vi "AudioTest.SoundCheck Data Log Graph Window - Composite.vi"() -> ()   [LabVIEW 2018]
uses:
  TypeDefs/AudioTest.Analysis Data Record.ctl
  <vilib>/KATE/Queues/Queue Utils.lvlib
panel:
  in  "Main Tab":enum32{"Data", "Setup"}(tab)
  in  "Snapshot":bool
  out "Name 1 1":string
  out "Graph1 1":cluster{"X":dbl[], "Y":dbl[]}[](graph)
  out "Graph1 2":cluster{"X":dbl[], "Y":dbl[]}[](graph)
  out "Name 1 2":string
  out "Name 3 3":string
  out "Graph3 3":cluster{"X":dbl[], "Y":dbl[]}[](graph)
  out "Name 3 2":string
  out "Graph3 2":cluster{"X":dbl[], "Y":dbl[]}[](graph)
  out "Name 3 1":string
  out "Graph3 1":cluster{"X":dbl[], "Y":dbl[]}[](graph)
  out "Name 2 4":string
  out "Graph2 4":cluster{"X":dbl[], "Y":dbl[]}[](graph)
  out "Graph2 3":cluster{"X":dbl[], "Y":dbl[]}[](graph)
  out "Name 2 3":string
  out "Graph2 2":cluster{"X":dbl[], "Y":dbl[]}[](graph)
  out "Name 2 2":string
  out "Graph2 1":cluster{"X":dbl[], "Y":dbl[]}[](graph)
  out "Name 2 1":string
  out "Graph1 4":cluster{"X":dbl[], "Y":dbl[]}[](graph)
  out "Name 1 4":string
  out "Graph1 3":cluster{"X":dbl[], "Y":dbl[]}[](graph)
  out "Name 1 3":string
  in  "Graphs":T1[](array[typedef])
  in  "QName":string="Plot_Composite"
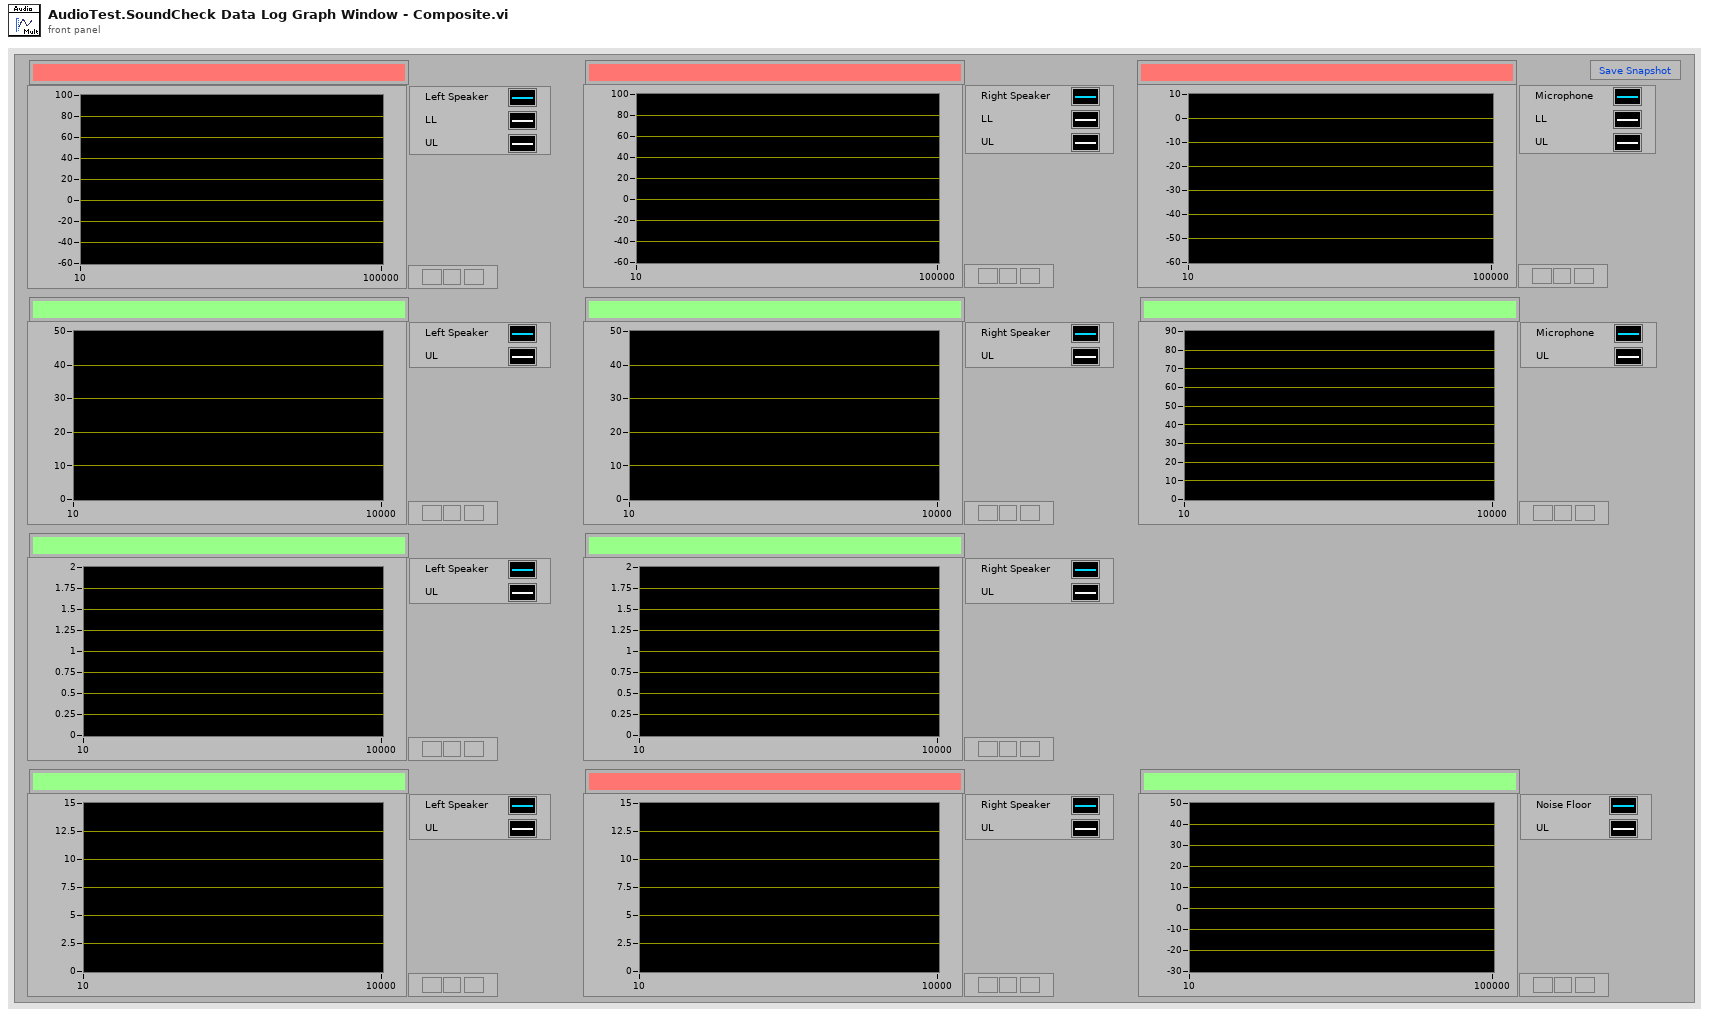
[diagram p1: front panel]
types:
  T1 = typedef "AudioTest.Analysis Data Record.ctl" = cluster{"Name":string, "X Units":string, "Y Units":string, "DataPlots":cluster{"X":dbl[], "Y":dbl[]}[], "LimitPlots":cluster{"X":dbl[], "Y":dbl[]}[], "DataPlotNames":string[], "LimitPlotNames":string[], "Fail":bool}
  T2 = typedef "imagedata.ctl" = cluster{"image type":i32, "image depth":i32, "image":u8[], "mask":u8[], "colors":u32[], "Rectangle":cluster{"left":i16, "top":i16, "right":i16, "bottom":i16}}
  T3 = enum32{"Invalid", "Standard", "Closed", "Hidden", "Minimized", "Maximized"}
  T4 = cluster{"Graphs":T1[], "PlotColors":u32[], "LimColors":u32[]}
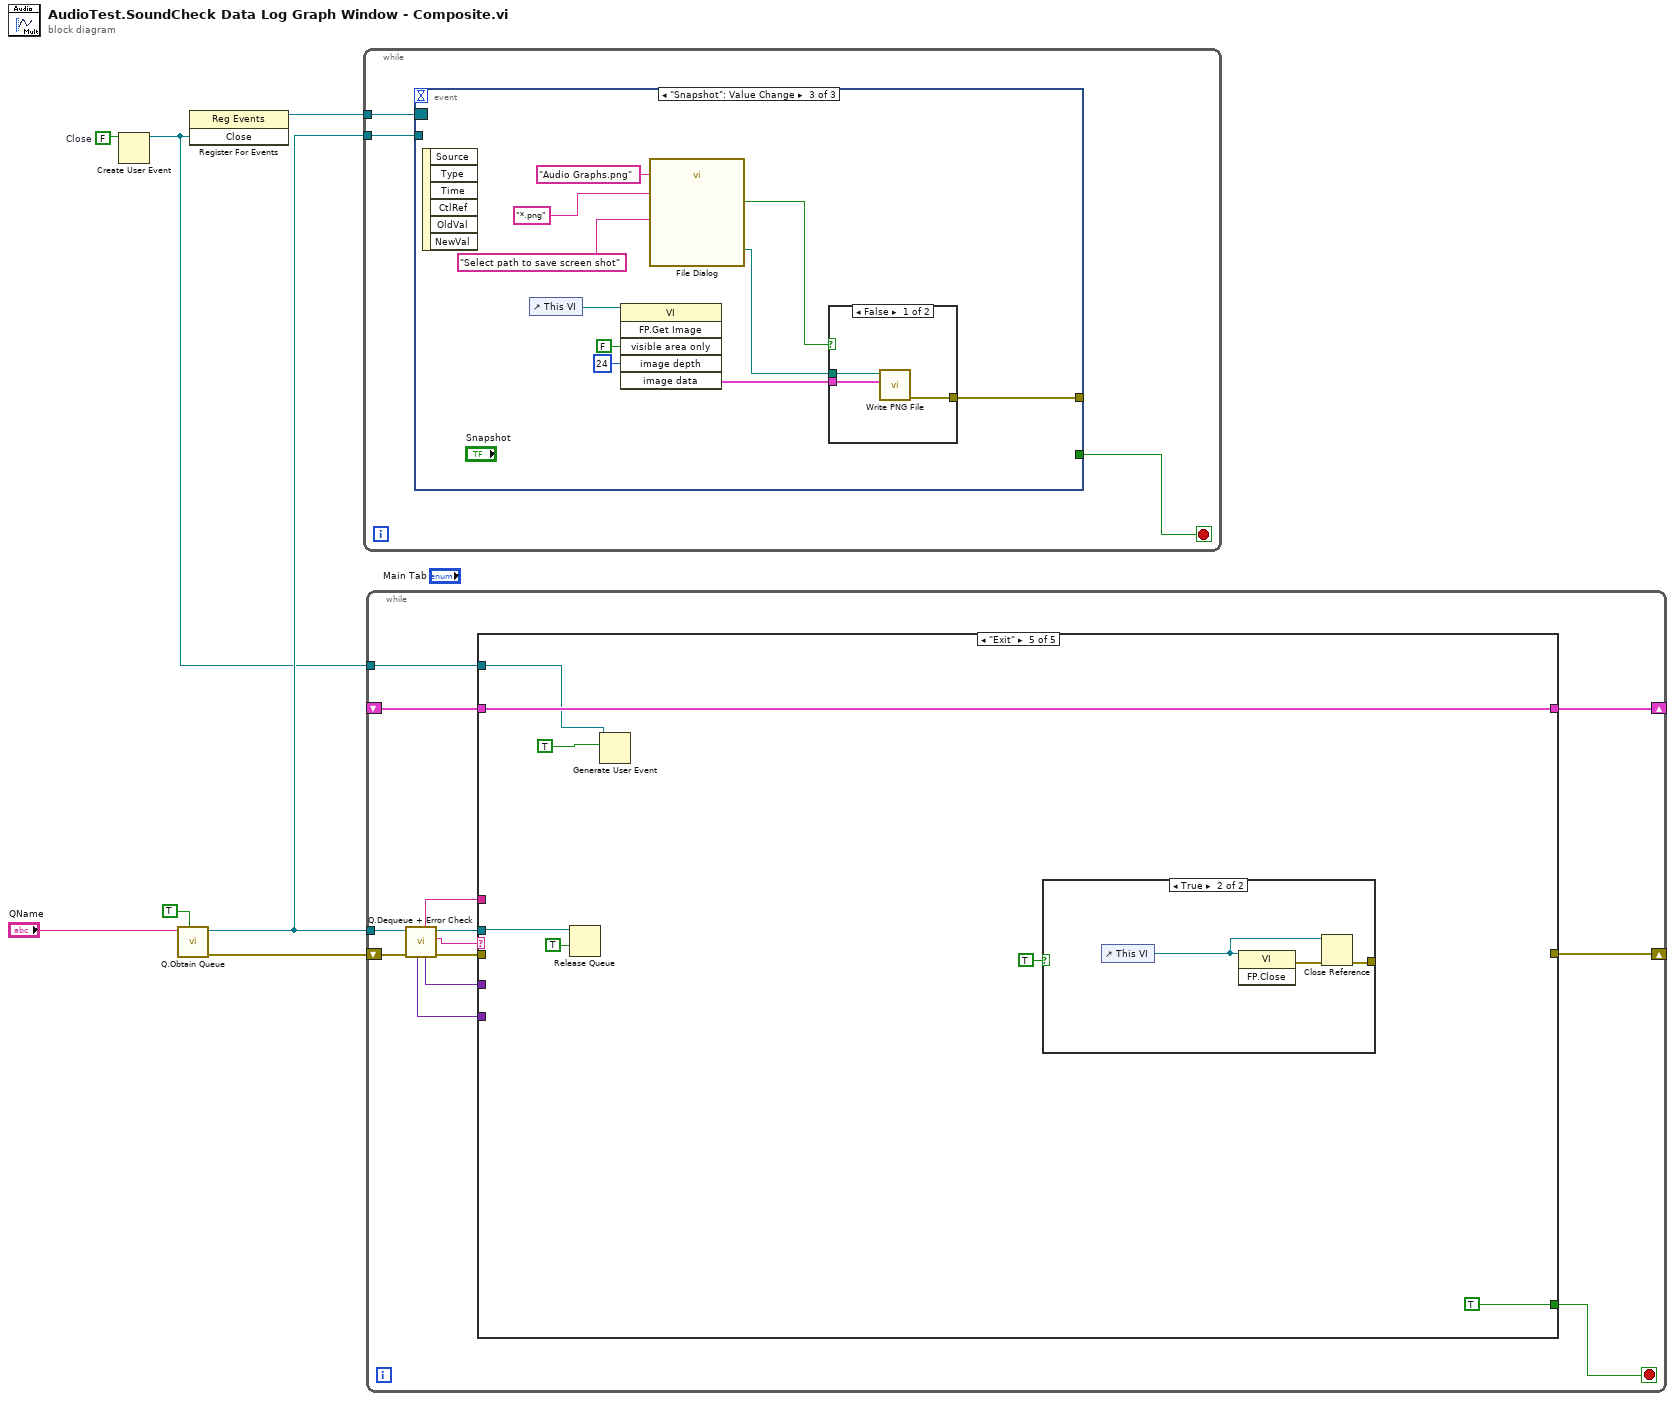
[diagram p0: block diagram]
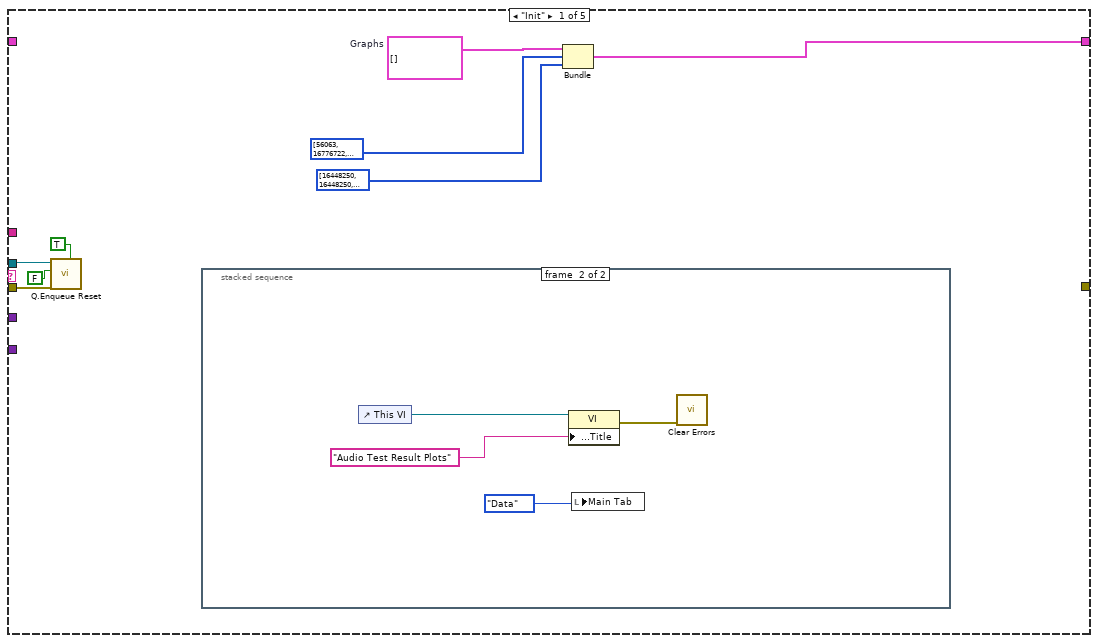
[diagram p2: hidden frame]
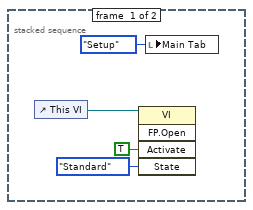
[diagram p3: hidden frame]
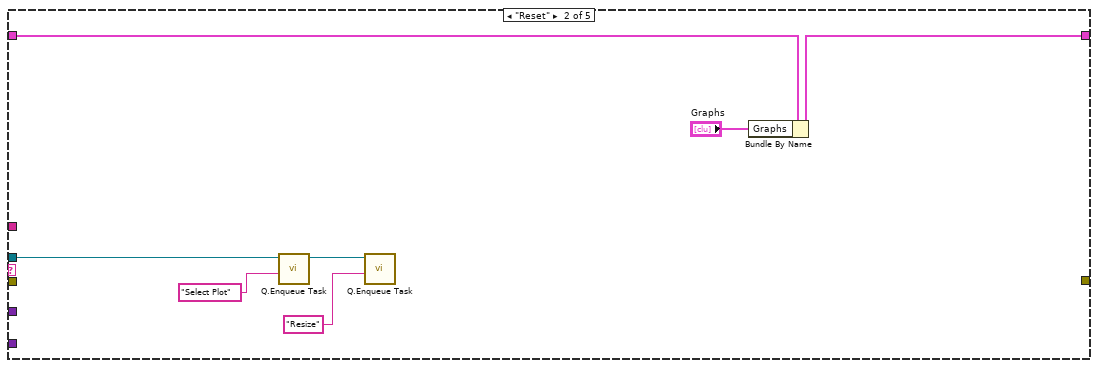
[diagram p4: hidden frame]
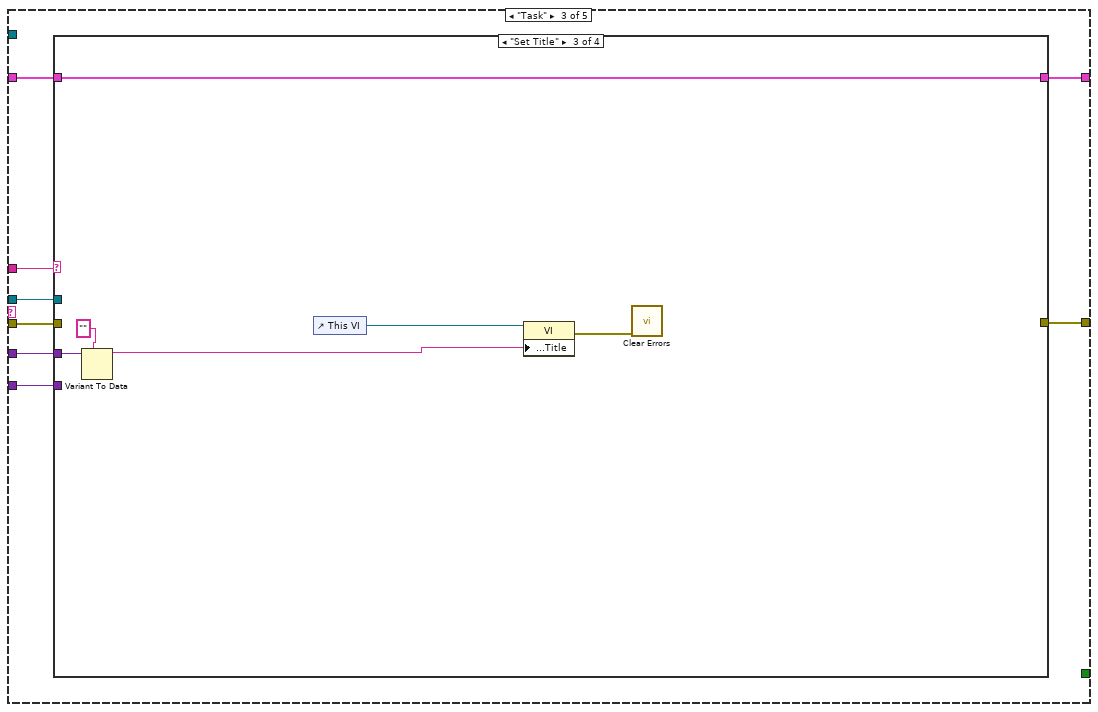
[diagram p5: hidden frame]
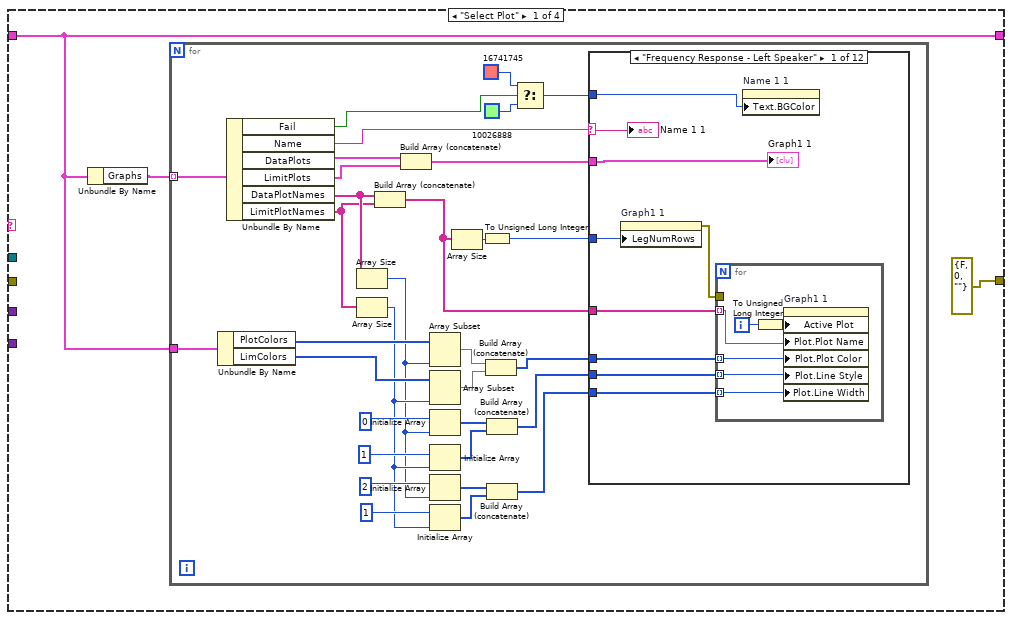
[diagram p6: hidden frame]
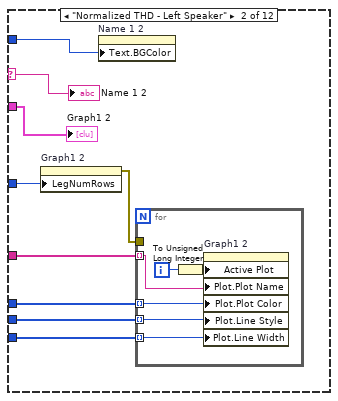
[diagram p7: hidden frame]
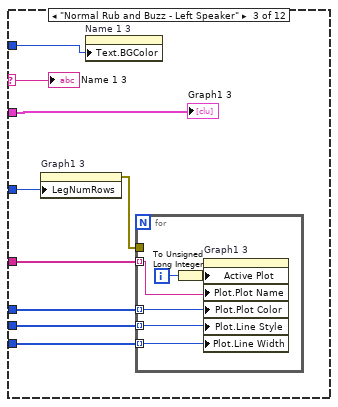
[diagram p8: hidden frame]
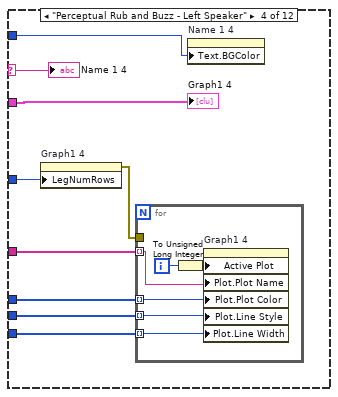
[diagram p9: hidden frame]
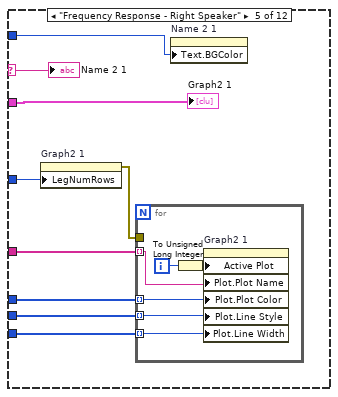
[diagram p10: hidden frame]
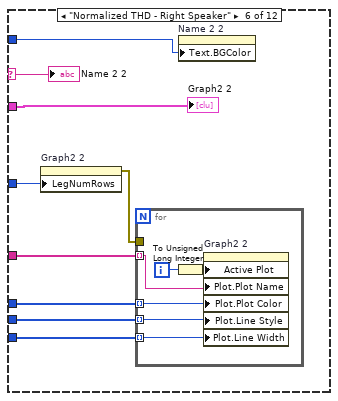
[diagram p11: hidden frame]
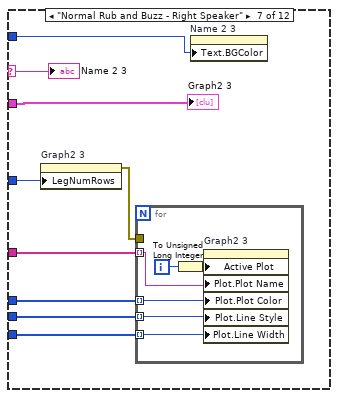
[diagram p12: hidden frame]
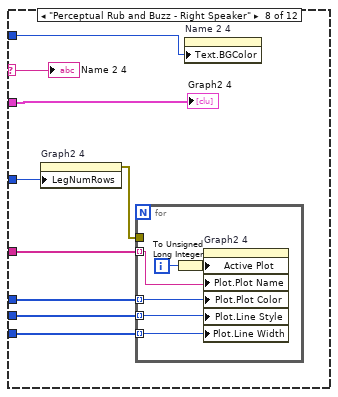
[diagram p13: hidden frame]
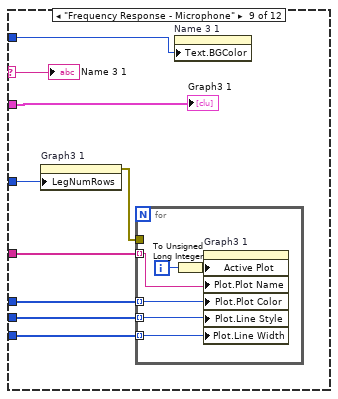
[diagram p14: hidden frame]
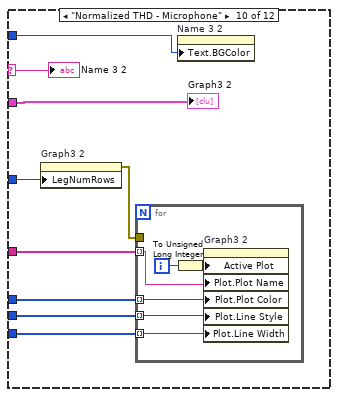
[diagram p15: hidden frame]
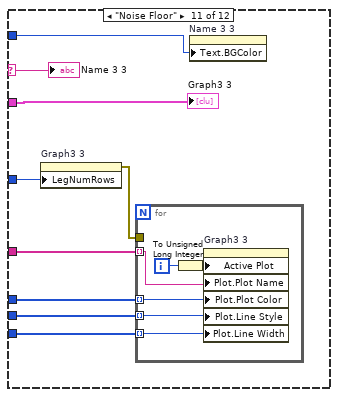
[diagram p16: hidden frame]
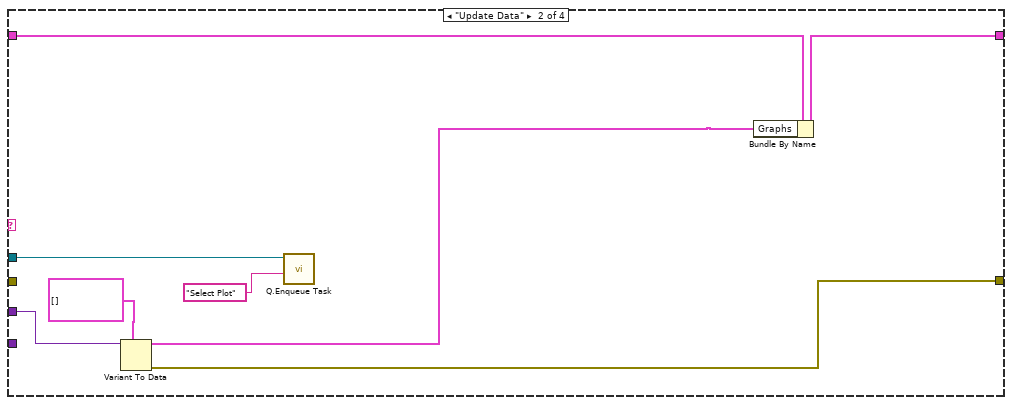
[diagram p18: hidden frame]
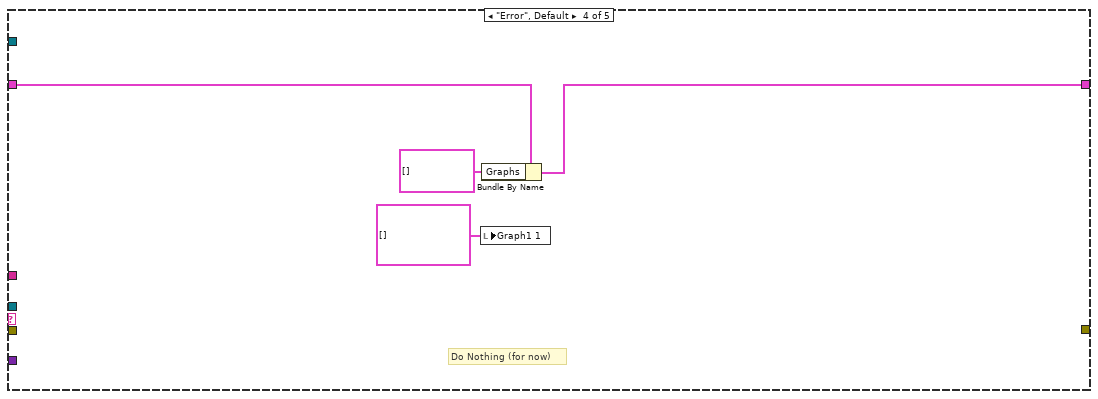
[diagram p20: hidden frame]
diagram:
  w7 = FALSE  # Close
  n1 = Create User Event(user event datatype=w7) -> (user event=w2:refnum<user-event>)  [unwired: 1 in, 1 out]
  n2 = call <vilib>:"Q.Obtain Queue.vi"("Enqueue Init"=TRUE, "Q Name"="QName") -> ("error out"=w4:errorcluster, "Q Out"=w3:refnum<queue>)  [unwired: 7 in, 1 out]
  n3 = register-events(w2) -> (reference out=w6:refnum<event-registration>)  [unwired: 2 in, 1 out]
  n4 = while {
    tunnel: w6 -> [w10]
    tunnel: w3 -> [w9]
    stop <- w8 stop-if-true
    n5 = event shown="[2] \"Snapshot\": Value Change" {
      selector: w10 -> [_ _ _]
      dyn-events: _ -> [_ _ _]
      timeout: _ -> [_ _ _]
      tunnel: w9 -> [w13 w16 _]
      tunnel: [TRUE TRUE _] -> w8
      tunnel: [_ _ w23] -> _
      event Panel Close? {
        n6 = event-data() -> ()  [unwired: 1 in, 4 out]
        n7 = call <vilib>:"Q.Enqueue Exit.vi"("Q In"=w13) -> ("error out"=w12:errorcluster)  [unwired: 9 in, 1 out]
        n8 = call <vilib>:"Clear Errors.vi"("error in (no error)"=w12) -> ()  [unwired: 5 in, 2 out]
        n9 = event-data("Discard?"=TRUE) -> ()  [unwired: 1 in, 1 out]
      }
      event User Event {
        n10 = event-data() -> ()  [unwired: 1 in, 4 out]
        n11 = call <vilib>:"Q.Enqueue Exit.vi"("Q In"=w16) -> ("error out"=w15:errorcluster)  [unwired: 9 in, 1 out]
        n12 = call <vilib>:"Clear Errors.vi"("error in (no error)"=w15) -> ()  [unwired: 5 in, 2 out]
      }
      event "Snapshot": Value Change {
        n13 = event-data() -> ()  [unwired: 1 in, 6 out]
        n14 = control-ref of="This VI"() -> (w27:refnum<vi>)
        n15 = invoke class="VI" method="FP.Get Image"(reference=w27, "visible area only"=FALSE ("Visible Area Only"), "image depth"=24 ("Image Depth")) -> ("image data"=w24:T2)  [unwired: 3 in, 5 out]
        n16 = call "File Dialog"("prompt"="Select path to save screen shot", "default name"="Audio Graphs.png", "pattern (all files)"="*.png") -> ("selected path"=w22:path, "cancelled"=w18:bool)  [unwired: 9 in, 2 out]
        n17 = case shown="False" w18 {
          tunnel: w24 -> [w30 _]
          tunnel: [w29 _] -> w23
          tunnel: w22 -> [w28 _]
          frame False {
            n18 = call <vilib>:"Write PNG File.vi"("image data"=w30, "path to PNG file"=w28) -> ("error out"=w29:errorcluster)  [unwired: 8 in, 1 out]
          }
          frame True {
          }
        }
      }
    }
  }
  n19 = while {
    shift-right: [w35] -> _
    shift-left: w4 -> [w40]
    tunnel: w3 -> [w38]
    shift-right: [w33] -> _
    shift-left: _ -> [w32]
    tunnel: w2 -> [w31]
    stop <- w34 stop-if-true
    n20 = call <vilib>:"Q.Dequeue + Error Check.vi"("Error In"=w40, "Q In"=w38) -> ("error out"=w41:errorcluster, "Cmd"=w43:string, "Q Out"=w42:refnum<queue>, "Data1"=w37:variant, "Sub"=w39:string, "Data2"=w36:variant)  [unwired: 4 in]
    n21 = case shown="\"Exit\"" w43 {
      tunnel: w42 -> [w51 w64 w73 _ w295]
      tunnel: w41 -> [w50 _ w72 _ _]
      tunnel: w39 -> [_ _ w74 _ _]
      tunnel: w37 -> [_ _ w71 _ _]
      tunnel: w36 -> [_ _ w70 _ _]
      tunnel: [_ _ w67 _ _] -> w35
      tunnel: [_ _ _ _ TRUE] -> w34
      tunnel: [w45 w66 w68 w292 w299] -> w33
      tunnel: w32 -> [_ w65 w69 w293 w299]
      tunnel: w31 -> [_ _ _ _ w298]
      frame "Init" {
        w48 = T1[] []  # Graphs
        n22 = call <vilib>:"Q.Enqueue Reset.vi"("Top of Q(T)"=TRUE, "Error In"=w50, "Flush Queue(T)"=FALSE, "Q In"=w51) -> ()  [unwired: 6 in, 2 out]
        n23 = stacked-sequence {
          frame #0 {
            n24 = control-ref of="This VI"() -> (w55:refnum<vi>)
            n25 = invoke class="VI" method="FP.Open"(reference=w55, "Activate"=TRUE ("Activate?"), "State"=T3."Standard") -> ()  [unwired: 2 in, 5 out]
            n26 = local write "Main Tab"(enum32{"Data", "Setup"}."Setup" ("Main Tab")) -> ()
          }
          frame #1 {
            n27 = control-ref of="This VI"() -> (w59:refnum<vi>)
            n28 = property class="VI"(reference=w59, "Front Panel.Title"="Audio Test Result Plots") -> (error out=w58:errorcluster)  [unwired: 1 in, 1 out]
            n29 = local write "Main Tab"(enum32{"Data", "Setup"}."Data" ("Main Tab")) -> ()
            n30 = call <vilib>:"Clear Errors.vi"("error in (no error)"=w58) -> ()  [unwired: 5 in, 2 out]
          }
        }
        n31 = Bundle("Graphs"=w48, "PlotColors"=u32[] [56063, 16776722, 16730898, 16711925, 6618880], "LimColors"=u32[] [16448250, 16448250, 16448250, 16448250, 16448250, 16448250]) -> (w45:T4)  [unwired: 1 in]
      }
      frame "Reset" {
        n32 = call <vilib>:"Q.Enqueue Task.vi"("Task Name"="Select Plot", "Q In"=w64) -> ("Q Out"=w61:refnum<queue>)  [unwired: 8 in, 1 out]
        n33 = call <vilib>:"Q.Enqueue Task.vi"("Task Name"="Resize", "Q In"=w61) -> ()  [unwired: 8 in, 2 out]
        n34 = Bundle By Name(cluster=w65, "Graphs"="Graphs") -> (w66:T4)
      }
      frame "Task" {
        n35 = case shown="\"Set Title\"" w74 {
          tunnel: w73 -> [_ w281 _ _]
          tunnel: w72 -> [_ _ _ _]
          tunnel: w71 -> [_ w278 w285 _]
          tunnel: w70 -> [_ _ _ _]
          tunnel: w69 -> [w77 w280 w288 w289]
          tunnel: [w77 w279 w288 w289] -> w68
          tunnel: [errorcluster {"status"=FALSE, "code"=0, "source"=""} ("error constant") w277 _ _] -> w67
          frame "Select Plot" {
            n36 = Unbundle By Name(w77) -> ("Graphs"=w75:T1[])
            n37 = for {
              tunnel: w77 -> [w104]
              tunnel: w75 -> [w83] mode=indexing
              n38 = Unbundle By Name(w104) -> ("PlotColors"=w101:u32[], "LimColors"=w100:u32[])
              n39 = Unbundle By Name(w83) -> ("Fail"=w79:bool, "Name"=w82:string, "DataPlots"=w109:cluster{"X":dbl[], "Y":dbl[]}[], "LimitPlots"=w108:cluster{"X":dbl[], "Y":dbl[]}[], "DataPlotNames"=w103:string[], "LimitPlotNames"=w102:string[])
              n40 = Array Size(array=w103) -> (size(s)=w86:i32)
              n41 = Array Size(array=w102) -> (size(s)=w87:i32)
              n42 = Build Array (concatenate)(w103, w102) -> (w105:string[])
              n43 = Build Array (concatenate)(w109, w108) -> (w84:cluster{"X":dbl[], "Y":dbl[]}[])
              n44 = Array Subset(array=w101, length=w86) -> (w99:u32[])  [unwired: 1 in]
              n45 = Array Subset(array=w100, length=w87) -> (w98:u32[])  [unwired: 1 in]
              n46 = Initialize Array(u8 0 ("Plot.Line Style"), w86) -> (w94:u8[])
              n47 = Initialize Array(u8 1 ("Plot.Line Style"), w87) -> (w93:u8[])
              n48 = Initialize Array(u8 2 ("Plot.Line Style"), w86) -> (w90:u8[])
              n49 = Initialize Array(u8 1 ("Plot.Line Style"), w87) -> (w91:u8[])
              n50 = Array Size(array=w105) -> (size(s)=w107:i32)
              n51 = To Unsigned Long Integer(number=w107) -> (unsigned 32bit integer=w106:u32)
              n52 = Build Array (concatenate)(w99, w98) -> (w97:u32[])
              n53 = Build Array (concatenate)(w94, w93) -> (w92:u8[])
              n54 = Build Array (concatenate)(w90, w91) -> (w85:u8[])
              n55 = Select(t=u32 16741745, s=w79, f=u32 10026888) -> (s? t:f=w78:u32)
              n56 = case shown="\"Frequency Response - Left Speaker\"" w82 {
                selector: w82 -> [w111 w126 w141 w156 w171 w186 w201 w216 w231 w246 w261 _]
                tunnel: w106 -> [w118 w133 w148 w163 w178 w193 w208 w223 w238 w253 w268 _]
                tunnel: w105 -> [w116 w131 w146 w161 w176 w191 w206 w221 w236 w251 w266 _]
                tunnel: w97 -> [w115 w130 w145 w160 w175 w190 w205 w220 w235 w250 w265 _]
                tunnel: w92 -> [w114 w129 w144 w159 w174 w189 w204 w219 w234 w249 w264 _]
                tunnel: w85 -> [w113 w128 w143 w158 w173 w188 w203 w218 w233 w248 w263 _]
                tunnel: w84 -> [w112 w127 w142 w157 w172 w187 w202 w217 w232 w247 w262 _]
                tunnel: w78 -> [w110 w125 w140 w155 w170 w185 w200 w215 w230 w245 w260 _]
                frame "Frequency Response - Left Speaker" {
                  n57 = property on="Graph1 1" class="XYGraph (strict)"("LegNumRows"=w118) -> (error out=w117:errorcluster)  [unwired: 2 in, 1 out]
                  n58 = for {
                    tunnel: w116 -> [w122] mode=indexing
                    tunnel: w117 -> [_]
                    tunnel: w115 -> [w121] mode=indexing
                    tunnel: w114 -> [w120] mode=indexing
                    tunnel: w113 -> [w119] mode=indexing
                    i -> [w123]
                    n59 = To Unsigned Long Integer(number=w123) -> (unsigned 32bit integer=w124:u32)
                    n60 = property on="Graph1 1" class="XYGraph (strict)"("Active Plot"=w124, "Plot.Plot Name"=w122, "Plot.Plot Color"=w121, "Plot.Line Style"=w120, "Plot.Line Width"=w119) -> ()  [unwired: 2 in, 2 out]
                  }
                  n61 = property on="Name 1 1" class="Str"("Text.BGColor"=w110) -> ()  [unwired: 2 in, 2 out]
                  "Graph1 1" <- w112
                  "Name 1 1" <- w111
                }
                frame "Normalized THD - Left Speaker" {
                  n62 = property on="Graph1 2" class="XYGraph (strict)"("LegNumRows"=w133) -> (error out=w132:errorcluster)  [unwired: 2 in, 1 out]
                  n63 = property on="Name 1 2" class="Str"("Text.BGColor"=w125) -> ()  [unwired: 2 in, 2 out]
                  n64 = for {
                    tunnel: w131 -> [w137] mode=indexing
                    tunnel: w132 -> [_]
                    tunnel: w130 -> [w136] mode=indexing
                    tunnel: w129 -> [w135] mode=indexing
                    tunnel: w128 -> [w134] mode=indexing
                    i -> [w138]
                    n65 = To Unsigned Long Integer(number=w138) -> (unsigned 32bit integer=w139:u32)
                    n66 = property on="Graph1 2" class="XYGraph (strict)"("Active Plot"=w139, "Plot.Plot Name"=w137, "Plot.Plot Color"=w136, "Plot.Line Style"=w135, "Plot.Line Width"=w134) -> ()  [unwired: 2 in, 2 out]
                  }
                  "Graph1 2" <- w127
                  "Name 1 2" <- w126
                }
                frame "Normal Rub and Buzz - Left Speaker" {
                  n67 = property on="Graph1 3" class="XYGraph (strict)"("LegNumRows"=w148) -> (error out=w147:errorcluster)  [unwired: 2 in, 1 out]
                  n68 = property on="Name 1 3" class="Str"("Text.BGColor"=w140) -> ()  [unwired: 2 in, 2 out]
                  n69 = for {
                    tunnel: w146 -> [w152] mode=indexing
                    tunnel: w147 -> [_]
                    tunnel: w145 -> [w151] mode=indexing
                    tunnel: w144 -> [w150] mode=indexing
                    tunnel: w143 -> [w149] mode=indexing
                    i -> [w153]
                    n70 = To Unsigned Long Integer(number=w153) -> (unsigned 32bit integer=w154:u32)
                    n71 = property on="Graph1 3" class="XYGraph (strict)"("Active Plot"=w154, "Plot.Plot Name"=w152, "Plot.Plot Color"=w151, "Plot.Line Style"=w150, "Plot.Line Width"=w149) -> ()  [unwired: 2 in, 2 out]
                  }
                  "Graph1 3" <- w142
                  "Name 1 3" <- w141
                }
                frame "Perceptual Rub and Buzz - Left Speaker" {
                  n72 = property on="Graph1 4" class="XYGraph (strict)"("LegNumRows"=w163) -> (error out=w162:errorcluster)  [unwired: 2 in, 1 out]
                  n73 = for {
                    tunnel: w161 -> [w167] mode=indexing
                    tunnel: w162 -> [_]
                    tunnel: w160 -> [w166] mode=indexing
                    tunnel: w159 -> [w165] mode=indexing
                    tunnel: w158 -> [w164] mode=indexing
                    i -> [w168]
                    n74 = To Unsigned Long Integer(number=w168) -> (unsigned 32bit integer=w169:u32)
                    n75 = property on="Graph1 4" class="XYGraph (strict)"("Active Plot"=w169, "Plot.Plot Name"=w167, "Plot.Plot Color"=w166, "Plot.Line Style"=w165, "Plot.Line Width"=w164) -> ()  [unwired: 2 in, 2 out]
                  }
                  n76 = property on="Name 1 4" class="Str"("Text.BGColor"=w155) -> ()  [unwired: 2 in, 2 out]
                  "Graph1 4" <- w157
                  "Name 1 4" <- w156
                }
                frame "Frequency Response - Right Speaker" {
                  n77 = property on="Graph2 1" class="XYGraph (strict)"("LegNumRows"=w178) -> (error out=w177:errorcluster)  [unwired: 2 in, 1 out]
                  n78 = for {
                    tunnel: w176 -> [w182] mode=indexing
                    tunnel: w177 -> [_]
                    tunnel: w175 -> [w181] mode=indexing
                    tunnel: w174 -> [w180] mode=indexing
                    tunnel: w173 -> [w179] mode=indexing
                    i -> [w183]
                    n79 = To Unsigned Long Integer(number=w183) -> (unsigned 32bit integer=w184:u32)
                    n80 = property on="Graph2 1" class="XYGraph (strict)"("Active Plot"=w184, "Plot.Plot Name"=w182, "Plot.Plot Color"=w181, "Plot.Line Style"=w180, "Plot.Line Width"=w179) -> ()  [unwired: 2 in, 2 out]
                  }
                  n81 = property on="Name 2 1" class="Str"("Text.BGColor"=w170) -> ()  [unwired: 2 in, 2 out]
                  "Graph2 1" <- w172
                  "Name 2 1" <- w171
                }
                frame "Normalized THD - Right Speaker" {
                  n82 = property on="Graph2 2" class="XYGraph (strict)"("LegNumRows"=w193) -> (error out=w192:errorcluster)  [unwired: 2 in, 1 out]
                  n83 = for {
                    tunnel: w191 -> [w197] mode=indexing
                    tunnel: w192 -> [_]
                    tunnel: w190 -> [w196] mode=indexing
                    tunnel: w189 -> [w195] mode=indexing
                    tunnel: w188 -> [w194] mode=indexing
                    i -> [w198]
                    n84 = To Unsigned Long Integer(number=w198) -> (unsigned 32bit integer=w199:u32)
                    n85 = property on="Graph2 2" class="XYGraph (strict)"("Active Plot"=w199, "Plot.Plot Name"=w197, "Plot.Plot Color"=w196, "Plot.Line Style"=w195, "Plot.Line Width"=w194) -> ()  [unwired: 2 in, 2 out]
                  }
                  n86 = property on="Name 2 2" class="Str"("Text.BGColor"=w185) -> ()  [unwired: 2 in, 2 out]
                  "Graph2 2" <- w187
                  "Name 2 2" <- w186
                }
                frame "Normal Rub and Buzz - Right Speaker" {
                  n87 = property on="Graph2 3" class="XYGraph (strict)"("LegNumRows"=w208) -> (error out=w207:errorcluster)  [unwired: 2 in, 1 out]
                  n88 = for {
                    tunnel: w206 -> [w212] mode=indexing
                    tunnel: w207 -> [_]
                    tunnel: w205 -> [w211] mode=indexing
                    tunnel: w204 -> [w210] mode=indexing
                    tunnel: w203 -> [w209] mode=indexing
                    i -> [w213]
                    n89 = To Unsigned Long Integer(number=w213) -> (unsigned 32bit integer=w214:u32)
                    n90 = property on="Graph2 3" class="XYGraph (strict)"("Active Plot"=w214, "Plot.Plot Name"=w212, "Plot.Plot Color"=w211, "Plot.Line Style"=w210, "Plot.Line Width"=w209) -> ()  [unwired: 2 in, 2 out]
                  }
                  n91 = property on="Name 2 3" class="Str"("Text.BGColor"=w200) -> ()  [unwired: 2 in, 2 out]
                  "Graph2 3" <- w202
                  "Name 2 3" <- w201
                }
                frame "Perceptual Rub and Buzz - Right Speaker" {
                  n92 = property on="Graph2 4" class="XYGraph (strict)"("LegNumRows"=w223) -> (error out=w222:errorcluster)  [unwired: 2 in, 1 out]
                  n93 = for {
                    tunnel: w221 -> [w227] mode=indexing
                    tunnel: w222 -> [_]
                    tunnel: w220 -> [w226] mode=indexing
                    tunnel: w219 -> [w225] mode=indexing
                    tunnel: w218 -> [w224] mode=indexing
                    i -> [w228]
                    n94 = To Unsigned Long Integer(number=w228) -> (unsigned 32bit integer=w229:u32)
                    n95 = property on="Graph2 4" class="XYGraph (strict)"("Active Plot"=w229, "Plot.Plot Name"=w227, "Plot.Plot Color"=w226, "Plot.Line Style"=w225, "Plot.Line Width"=w224) -> ()  [unwired: 2 in, 2 out]
                  }
                  n96 = property on="Name 2 4" class="Str"("Text.BGColor"=w215) -> ()  [unwired: 2 in, 2 out]
                  "Graph2 4" <- w217
                  "Name 2 4" <- w216
                }
                frame "Frequency Response - Microphone" {
                  n97 = property on="Graph3 1" class="XYGraph (strict)"("LegNumRows"=w238) -> (error out=w237:errorcluster)  [unwired: 2 in, 1 out]
                  n98 = for {
                    tunnel: w236 -> [w242] mode=indexing
                    tunnel: w237 -> [_]
                    tunnel: w235 -> [w241] mode=indexing
                    tunnel: w234 -> [w240] mode=indexing
                    tunnel: w233 -> [w239] mode=indexing
                    i -> [w243]
                    n99 = To Unsigned Long Integer(number=w243) -> (unsigned 32bit integer=w244:u32)
                    n100 = property on="Graph3 1" class="XYGraph (strict)"("Active Plot"=w244, "Plot.Plot Name"=w242, "Plot.Plot Color"=w241, "Plot.Line Style"=w240, "Plot.Line Width"=w239) -> ()  [unwired: 2 in, 2 out]
                  }
                  n101 = property on="Name 3 1" class="Str"("Text.BGColor"=w230) -> ()  [unwired: 2 in, 2 out]
                  "Graph3 1" <- w232
                  "Name 3 1" <- w231
                }
                frame "Normalized THD - Microphone" {
                  n102 = property on="Graph3 2" class="XYGraph (strict)"("LegNumRows"=w253) -> (error out=w252:errorcluster)  [unwired: 2 in, 1 out]
                  n103 = for {
                    tunnel: w251 -> [w257] mode=indexing
                    tunnel: w252 -> [_]
                    tunnel: w250 -> [w256] mode=indexing
                    tunnel: w249 -> [w255] mode=indexing
                    tunnel: w248 -> [w254] mode=indexing
                    i -> [w258]
                    n104 = To Unsigned Long Integer(number=w258) -> (unsigned 32bit integer=w259:u32)
                    n105 = property on="Graph3 2" class="XYGraph (strict)"("Active Plot"=w259, "Plot.Plot Name"=w257, "Plot.Plot Color"=w256, "Plot.Line Style"=w255, "Plot.Line Width"=w254) -> ()  [unwired: 2 in, 2 out]
                  }
                  n106 = property on="Name 3 2" class="Str"("Text.BGColor"=w245) -> ()  [unwired: 2 in, 2 out]
                  "Graph3 2" <- w247
                  "Name 3 2" <- w246
                }
                frame "Noise Floor" {
                  n107 = property on="Graph3 3" class="XYGraph (strict)"("LegNumRows"=w268) -> (error out=w267:errorcluster)  [unwired: 2 in, 1 out]
                  n108 = for {
                    tunnel: w266 -> [w272] mode=indexing
                    tunnel: w267 -> [_]
                    tunnel: w265 -> [w271] mode=indexing
                    tunnel: w264 -> [w270] mode=indexing
                    tunnel: w263 -> [w269] mode=indexing
                    i -> [w273]
                    n109 = To Unsigned Long Integer(number=w273) -> (unsigned 32bit integer=w274:u32)
                    n110 = property on="Graph3 3" class="XYGraph (strict)"("Active Plot"=w274, "Plot.Plot Name"=w272, "Plot.Plot Color"=w271, "Plot.Line Style"=w270, "Plot.Line Width"=w269) -> ()  [unwired: 2 in, 2 out]
                  }
                  n111 = property on="Name 3 3" class="Str"("Text.BGColor"=w260) -> ()  [unwired: 2 in, 2 out]
                  "Graph3 3" <- w262
                  "Name 3 3" <- w261
                }
                frame Default {
                }
              }
            }
          }
          frame "Update Data" {
            n112 = Variant To Data(type=T1[] [] ("Graphs"), Variant=w278) -> (data=w276:T1[], error out=w277:errorcluster)  [unwired: 1 in]
            n113 = call <vilib>:"Q.Enqueue Task.vi"("Task Name"="Select Plot", "Q In"=w281) -> ()  [unwired: 8 in, 2 out]
            n114 = Bundle By Name(cluster=w280, "Graphs"=w276) -> (w279:T4)
          }
          frame "Set Title" {
            n115 = Variant To Data(type="", Variant=w285) -> (data=w283:string)  [unwired: 1 in, 1 out]
            n116 = control-ref of="This VI"() -> (w287:refnum<vi>)
            n117 = property class="VI"(reference=w287, "Front Panel.Title"=w283) -> (error out=w286:errorcluster)  [unwired: 1 in, 1 out]
            n118 = call <vilib>:"Clear Errors.vi"("error in (no error)"=w286) -> ()  [unwired: 5 in, 2 out]
          }
          frame Default {
          }
        }
      }
      frame "Error", Default {
        # "Do Nothing (for now)"
        n119 = local write "Graph1 1"(cluster{"X":dbl[], "Y":dbl[]}[] [] ("XY Graph")) -> ()
        n120 = Bundle By Name(cluster=w293, "Graphs"=T1[] []) -> (w292:T4)
      }
      frame "Exit" {
        n121 = Release Queue(queue=w295, force destroy? (F)=TRUE) -> ()  [unwired: 1 in, 3 out]
        n122 = Generate User Event(user event=w298, event data cluster=TRUE ("event data")) -> ()  [unwired: 2 in, 2 out]
        n123 = case shown="True" TRUE {
          tunnel: [_ w301] -> _
          frame False {
          }
          frame True {
            n124 = control-ref of="This VI"() -> (w303:refnum<vi>)
            n125 = invoke class="VI" method="FP.Close"(reference=w303) -> (error out=w302:errorcluster)  [unwired: 2 in, 2 out]
            n126 = Close Reference(reference=w303, error in (no error)=w302) -> (error out=w301:errorcluster)
          }
        }
      }
    }
  }
